vi "G#Object_ObjectToByteArray.vi"(1 "reference":refnum<class "G#Object.lvclass">, 5 "error in (no error)":errorcluster) -> (15 "unsigned byte array":u8[](array[numeric]), 19 "error out":errorcluster)   [LabVIEW 2017, in "G#Object.lvclass"]
uses:
  G#Object.lvclass
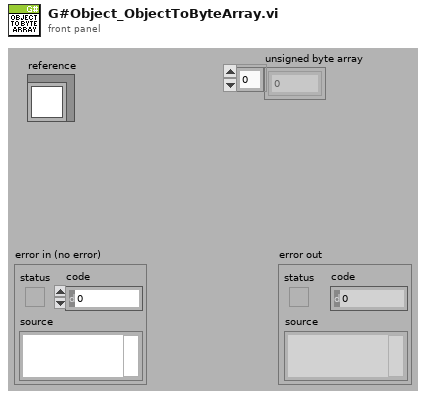
[diagram p1: front panel]
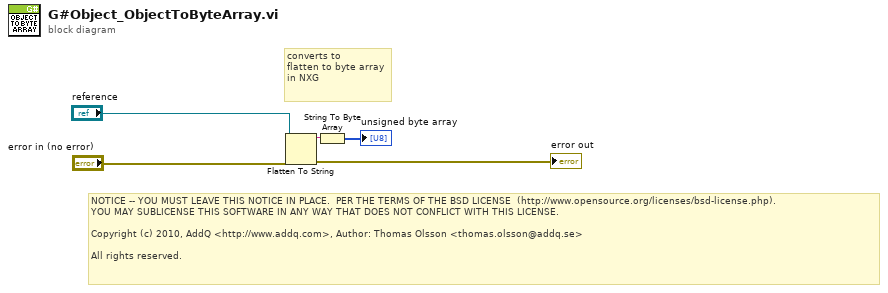
[diagram p0: block diagram]
diagram:
  # "converts to\nflatten to byte array\nin NXG"
  # "NOTICE -- YOU MUST LEAVE THIS NOTICE IN PLACE.  PER THE TERMS OF THE BSD LICENSE  (http://www.opensource.org/licenses/bsd-license.php).\nYOU MAY SUBLICENSE THIS SOFTWARE IN ANY WAY THAT DOES NOT CONFLICT WITH THIS LICENSE.\n\nCopyright (c) 2010, AddQ <http://www.addq.com>, Author: Thomas Olsson <thomas.olsson@addq.se>\n\nAll rights reserved."
  n1 = Flatten To String(anything="reference", error in (no error)="error in (no error)") -> (data string=w3:string, error out=→"error out":errorcluster)  [unwired: 2 in, 1 out]
  n2 = String To Byte Array(string=w3) -> (unsigned byte array=→"unsigned byte array":u8[])
